vi "Matrix_target.vi"() -> ()   [LabVIEW 2013]
uses:
  <vilib>/Platform/TimedLoop/XDataNode/wakeup.ctl
  <vilib>/Platform/TimedLoop/XDataNode/XDNodeRunTimeDep.lvlib
  <vilib>/Platform/TimedLoop/XDataNode/nitl_modes.ctl
  <vilib>/Platform/TimedLoop/XDataNode/timing_clust.ctl
  <vilib>/Platform/TimedLoop/XDataNode/XDataNode.xnode
  <vilib>/eio/EIONode/EIONode.xnode
  <vilib>/rvi/eio/common/nirviEmuTemplateMethod_errors.vi
  <vilib>/rvi/DataTransferAndStorage/Container/XNode/niFpgaContainer.xnode
  <vilib>/rvi/interface/RandomDataEmulation/nirviRandomDataFpgaReadWriteTemplate.vi
panel:
  out "READ_Number":u64
  in  "RESET":bool
  in  "55":i16
  in  "56":i16
  in  "75":i16
  in  "73":i16
  in  "57":i16=89
  out "String_counter":i16
  in  "String_number":i16
  in  "I2C_Write":bool
  in  "Read2":u8 format="%x"
  in  "Read1":u8 format="%x"
  in  "Device_Read":u8=187 format="%x"
  in  "Reg":u8=9 format="%x"
  in  "Device_Write":u8=186 format="%x"
  in  "91":i16=89
  in  "100_Sclk_divider":i32=25
  out "Sclk":bool
  in  "75_Stop":i16=75
  in  "53":i16=53
  in  "35":i16=35
  in  "17":i16=17
  in  "71":i16=71
  in  "54":i16=54
  in  "36":i16=36
  in  "18":i16=18
  in  "72":i16=72
  in  "50_Rise/Fall divider":i32=50
  in  "0_WE divider":i32
  in  "DataUp":u64
  in  "DataLow":u64
  out "ACK":bool[](array[boolean])
  out "Data_Array":bool[](array[boolean])
  in  "I2C_Request":bool
  in  "FALSE_LV":bool
  in  "FALSE_PIXCLK":bool
  in  "TRUE_FV":bool
  in  "Линия_ прочтена":bool
  in  "Остановите":bool
  out "Линия_готова_на_все":bool
  in  "Читай_Линию":bool
  in  "1_EXTCLK_divider":i16=2
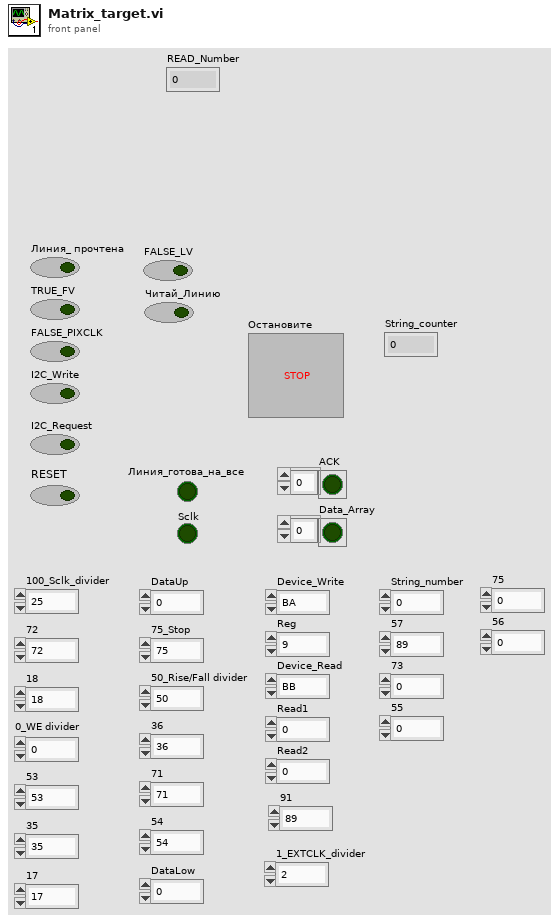
[diagram p1: front panel]
types:
  T1 = typedef "XDNodeRunTimeDep.lvlib/timing_clust.ctl" = cluster{"Expected End [f-1]":u64, "Actual End [f-1]":u64, "Finished Late? [f-1]":bool, "Expected End [i-1]":u64, "Actual End [i-1]":u64, "Finished Late? [i-1]":bool, "Expected Start [i]":u64, "Actual Start [i]":u64, "Expected Start [f]":u64, "Actual Start [f]":u64, "Source Name":string, "Structure Name":string, "Period":i64, "Deadline":i64, "Offset":i64, "Start":i64, "Priority":i32, "Timeout":i32, "Mode":T2, "Wakeup Reason":T3, "Error":errorcluster, "Source Type":string, "Secondary Source Type":string, "Global End Time":u64, "Global Start Time":u64, "Frame Duration":u64, "Iteration Duration":u64, "Assigned CPU":i32, "I/O Scan Engine Mode":u32}
  T2 = typedef "XDNodeRunTimeDep.lvlib/nitl_modes.ctl" = enum32{"No Change", "Process missed periods, maintain original phase", "Discard missed periods, maintain original phase", "Process missed periods, ignore original phase", "Discard missed periods, ignore original phase"}
  T3 = typedef "XDNodeRunTimeDep.lvlib/wakeup.ctl" = enum32{"Normal", "Aborted", "Asynchronous wakeup", "Timing source error", "Timed loop error", "Timeout"}
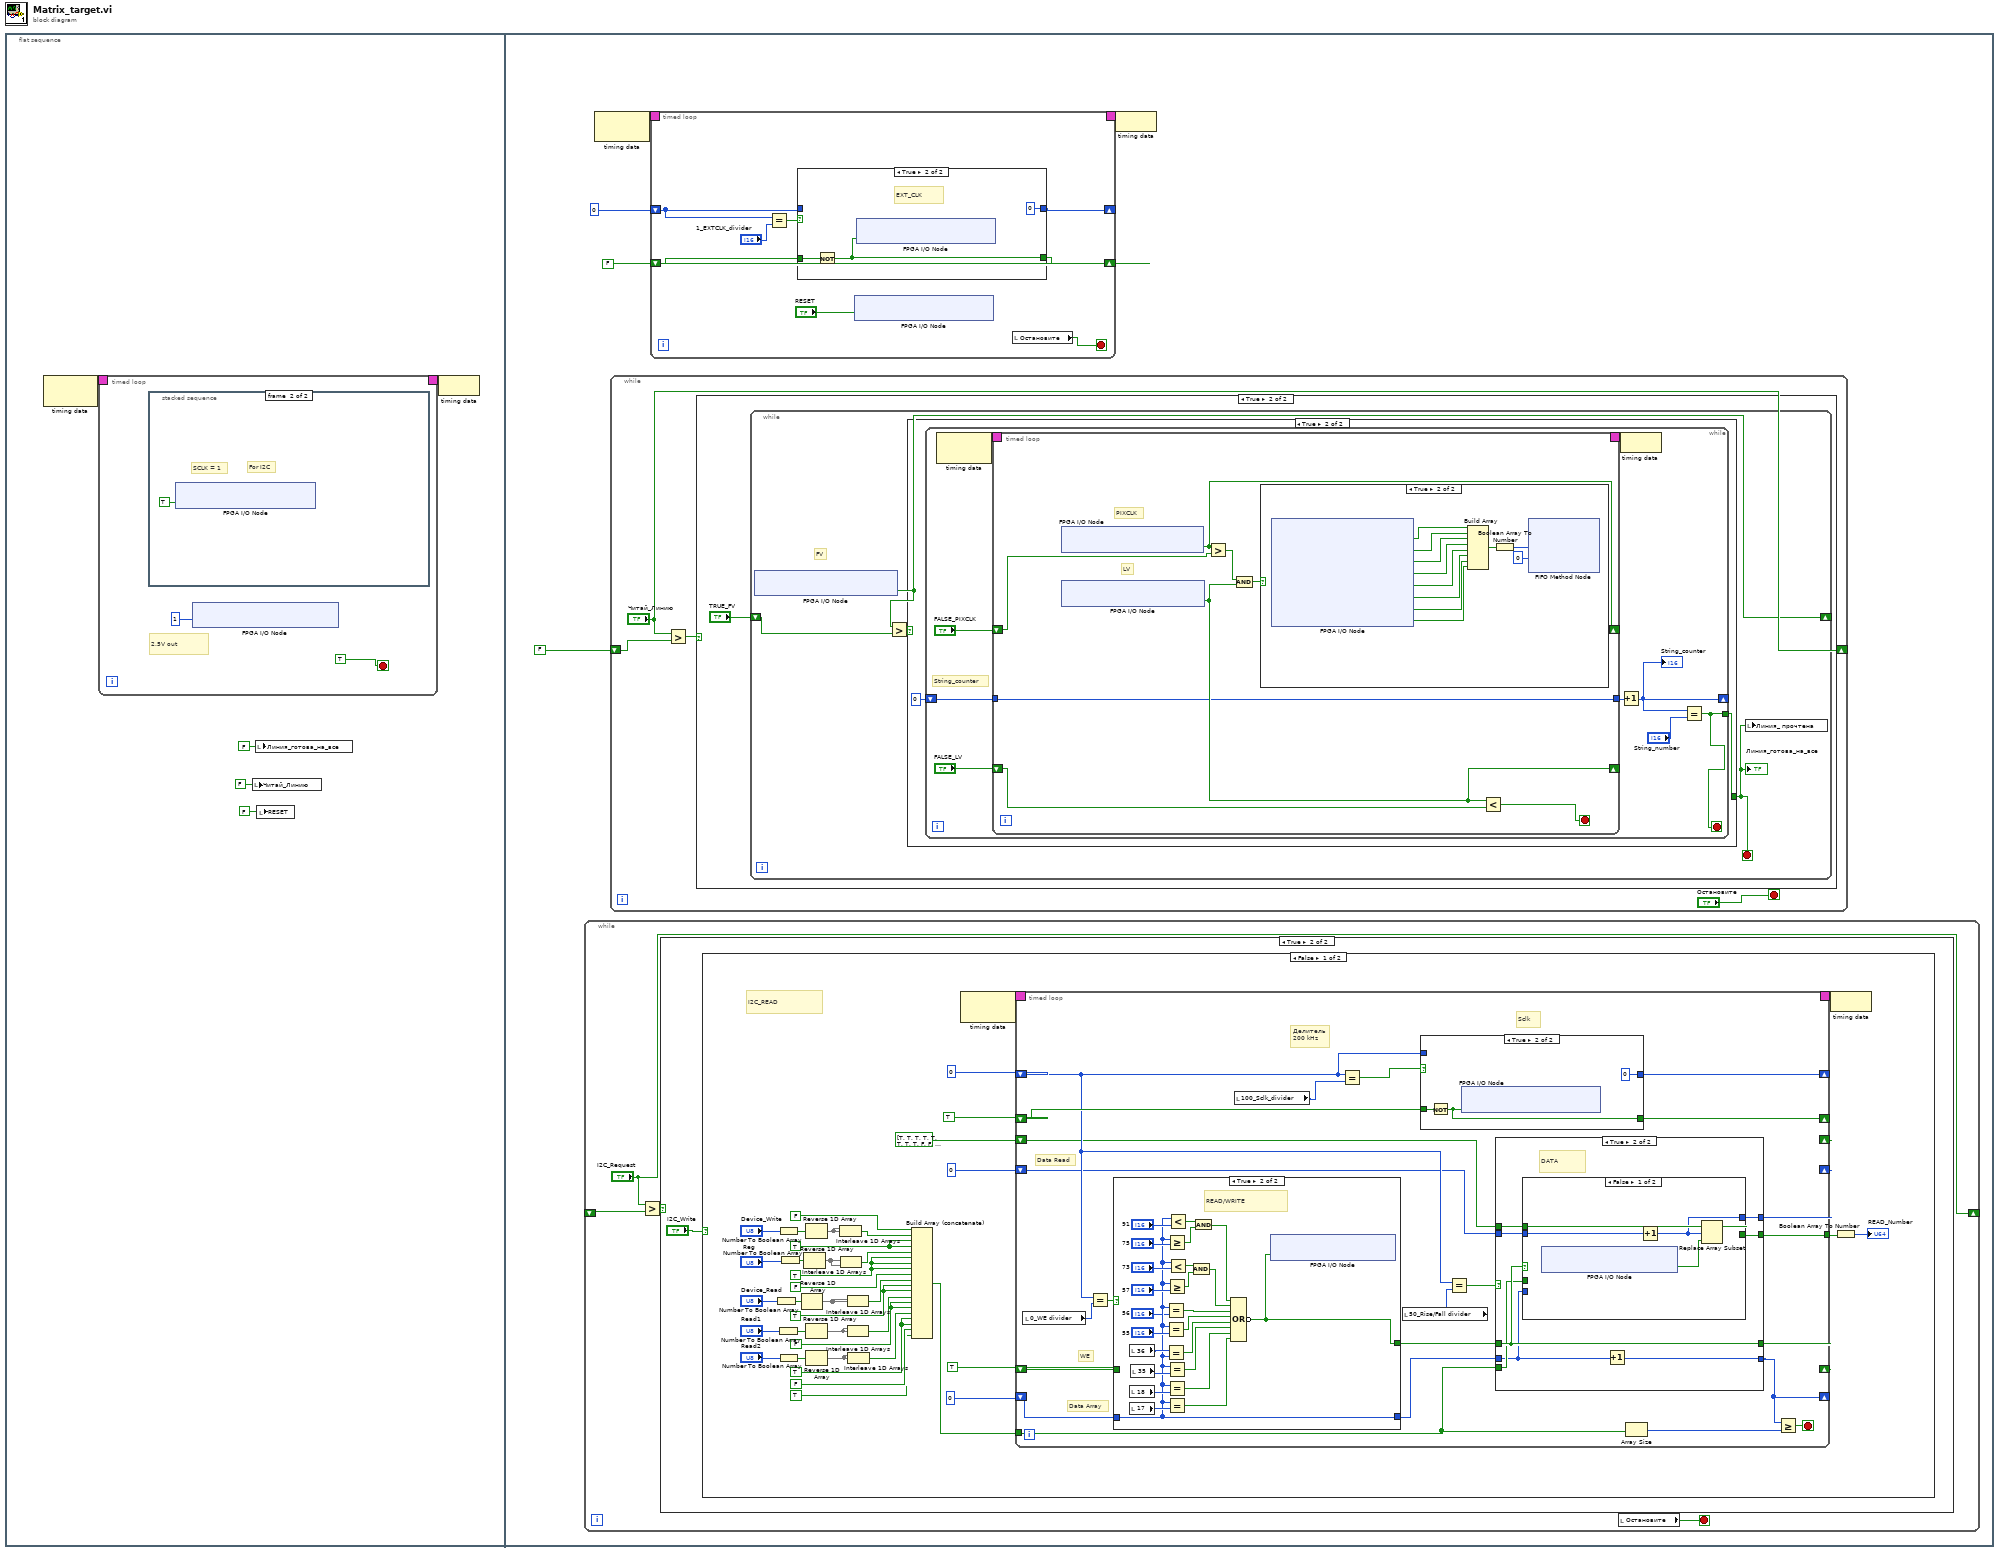
[diagram p0: block diagram]
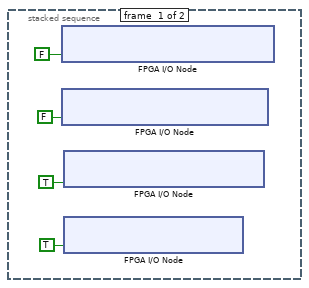
[diagram p2: hidden frame]
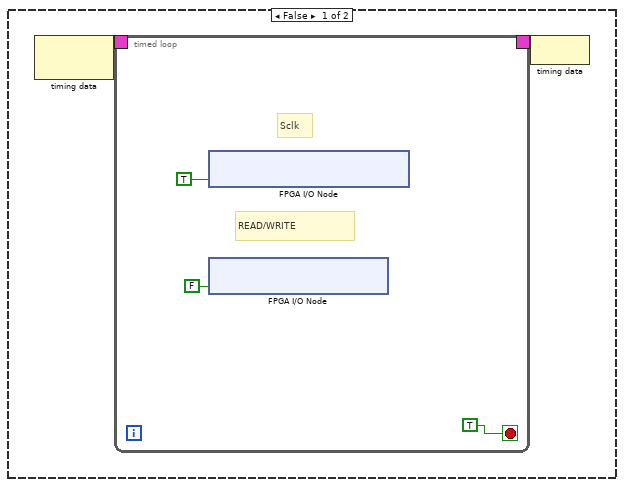
[diagram p3: hidden frame]
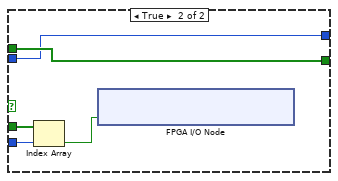
[diagram p6: hidden frame]
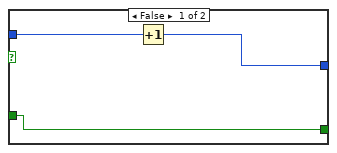
[diagram p7: hidden frame]
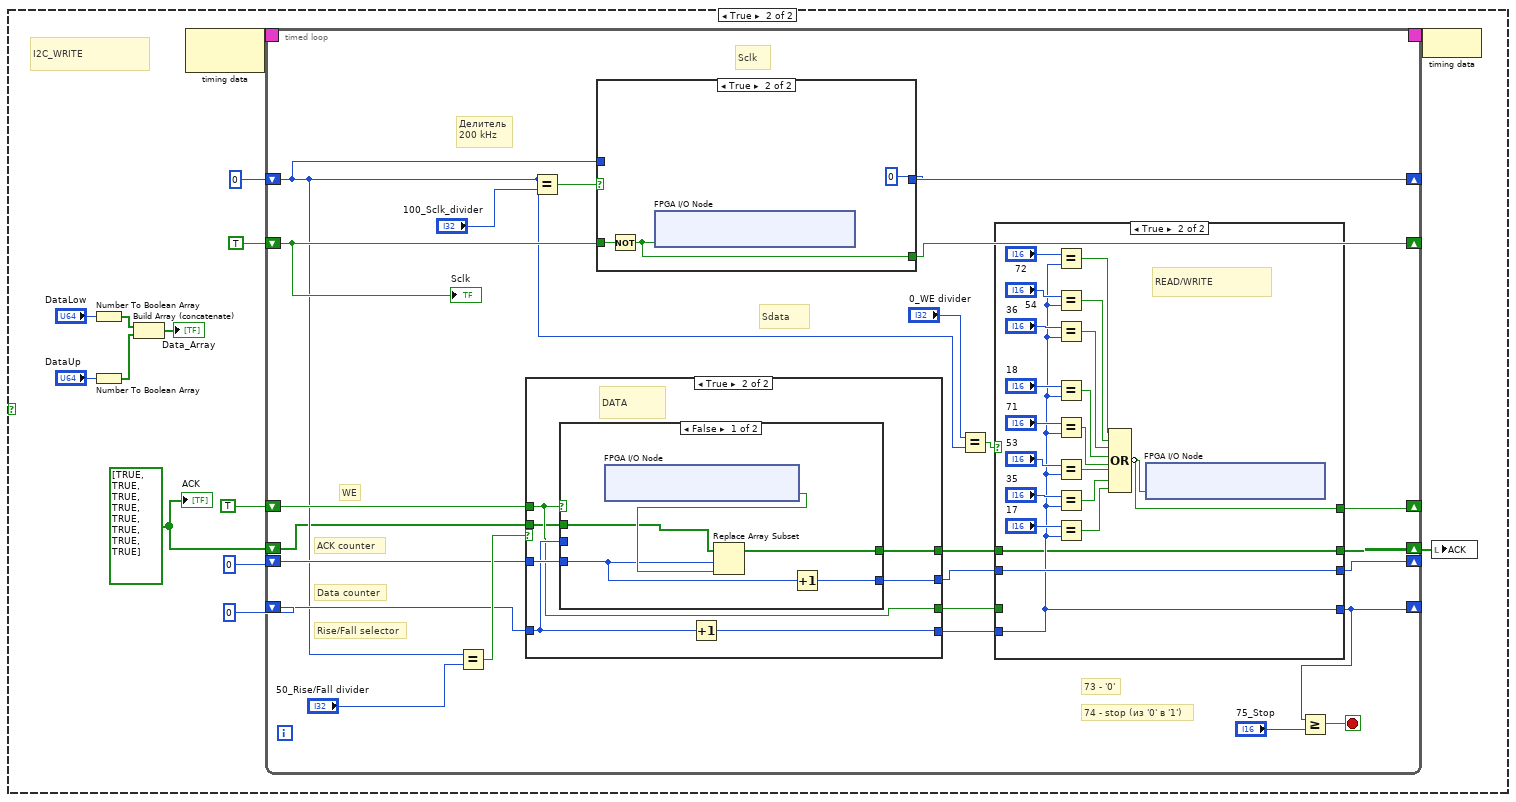
[diagram p8: hidden frame]
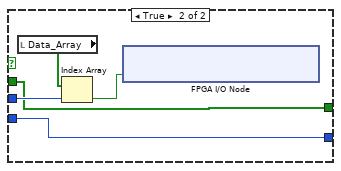
[diagram p11: hidden frame]
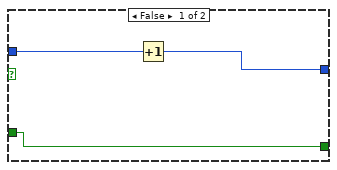
[diagram p12: hidden frame]
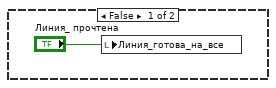
[diagram p13: hidden frame]
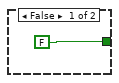
[diagram p14: hidden frame]
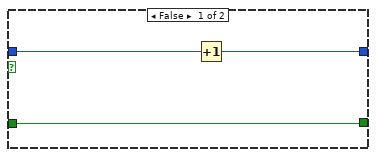
[diagram p16: hidden frame]
diagram:
  n1 = flat-sequence {
    frame #0 {
      n2 = node-c288() -> (w3:T1)  [unwired: 1 in]
      n3 = timed-loop {
        timing: w3 -> [_]
        timing-out: [_] -> w2
        stop <- TRUE stop-if-true
        # "2.5V out"
        n4 = stacked-sequence {
          frame #0 {
            n5 = xnode "FPGA I/O Node"("IO Module\\DDCA_DIO16-23_WE"=FALSE ("IO Module\\DDCA_DIO16-23_WE")) -> ()  [unwired: 1 in, 1 out]
            n6 = xnode "FPGA I/O Node"("IO Module\\DDCA_DIO8-15_WE"=FALSE ("IO Module\\DDCA_DIO8-15_WE")) -> ()  [unwired: 1 in, 1 out]
            n7 = xnode "FPGA I/O Node"("IO Module\\DDCA_DIO0-7_WE"=TRUE ("IO Module\\DDCA_DIO0-7_WE")) -> ()  [unwired: 1 in, 1 out]
            n8 = xnode "FPGA I/O Node"("IO Module\\DDCA_PFI_WE"=TRUE ("IO Module\\DDCA_DIO0-7_WE")) -> ()  [unwired: 1 in, 1 out]
          }
          frame #1 {
            # "For I2C"
            # "SCLK = 1"
            n9 = xnode "FPGA I/O Node"("IO Module\\DDCA_DIO6_Write"=TRUE ("IO Module\\DDCA_DIO6_Write")) -> ()  [unwired: 1 in, 1 out]
          }
        }
        n10 = xnode "FPGA I/O Node"("IO Module\\Local_Supply_Select"=u8 1 ("IO Module\\Local_Supply_Select")) -> ()  [unwired: 1 in, 1 out]
      }
      n11 = local write "Читай_Линию"(FALSE ("Читай_Линию")) -> ()
      n12 = local write "Линия_готова_на_все"(FALSE ("Линия_готова_на_все")) -> ()
      n13 = local write "RESET"(FALSE ("RESET")) -> ()
      n14 = node-c288(w2) -> ()
    }
    frame #1 {
      n15 = while {
        shift-right: ["I2C_Request"] -> _
        shift-left: _ -> [w25]
        stop <- w23 stop-if-true
        n16 = Greater?(x="I2C_Request", y=w25) -> (0:w24:bool)
        n17 = case shown="True" w24 {
          frame False {
            n18 = node-c288() -> (w27:T1)  [unwired: 1 in]
            n19 = timed-loop {
              timing: w27 -> [_]
              timing-out: [_] -> w26
              stop <- TRUE stop-if-true
              # "READ/WRITE"
              # "Sclk"
              n20 = xnode "FPGA I/O Node"("IO Module\\DDCA_DIO6_Write"=TRUE) -> ()  [unwired: 1 in, 1 out]
              n21 = xnode "FPGA I/O Node"("IO Module\\DDCA_PFI_WE"=FALSE ("IO Module\\DDCA_PFI_WE")) -> ()  [unwired: 1 in, 1 out]
            }
            n22 = node-c288(w26) -> ()
          }
          frame True {
            n23 = case shown="False" "I2C_Write" {
              frame False {
                w49 = TRUE
                w51 = FALSE
                w55 = TRUE
                w58 = TRUE
                w61 = TRUE
                # "I2C_READ"
                n24 = Number To Boolean Array(number="Device_Read") -> (Boolean array=w66:bool[])
                n25 = Number To Boolean Array(number="Read1") -> (Boolean array=w46:bool[])
                n26 = Number To Boolean Array(number="Device_Write") -> (Boolean array=w64:bool[])
                n27 = Number To Boolean Array(number="Read2") -> (Boolean array=w45:bool[])
                n28 = Number To Boolean Array(number="Reg") -> (Boolean array=w65:bool[])
                n29 = Reverse 1D Array(array=w66) -> (reversed array=w42:bool[])
                n30 = Reverse 1D Array(array=w65) -> (reversed array=w43:bool[])
                n31 = Reverse 1D Array(array=w64) -> (reversed array=w44:bool[])
                n32 = Reverse 1D Array(array=w46) -> (reversed array=w41:bool[])
                n33 = Reverse 1D Array(array=w45) -> (reversed array=w40:bool[])
                n34 = Interleave 1D Arrays(w44, w44) -> (w62:bool[])
                n35 = Interleave 1D Arrays(w43, w43) -> (w60:bool[])
                n36 = Interleave 1D Arrays(w42, w42) -> (w56:bool[])
                n37 = Interleave 1D Arrays(w41, w41) -> (w52:bool[])
                n38 = Interleave 1D Arrays(w40, w40) -> (w50:bool[])
                n39 = Build Array (concatenate)(FALSE, w62, w61, w61, w60, w58, w58, w58, FALSE, w56, w55, w55, w52, w51, w51, w50, w49, w49, FALSE, TRUE) -> (w59:bool[])
                n40 = node-c288() -> (w75:T1)  [unwired: 1 in]
                n41 = timed-loop {
                  timing: w75 -> [_]
                  timing-out: [_] -> w74
                  shift-right: [w95] -> _
                  shift-left: i16 0 -> [w89]
                  shift-right: [w96] -> _
                  shift-left: TRUE -> [w97]
                  shift-right: [w92] -> _
                  shift-left: TRUE -> [w94]
                  shift-right: [w84] -> _
                  shift-left: i16 0 -> [w88]
                  tunnel: w59 -> [w86]
                  shift-right: [w77] -> _
                  shift-left: bool[] [TRUE, TRUE, TRUE, TRUE, TRUE, TRUE, TRUE, TRUE, FALSE, FALSE, FALSE, FALSE, FALSE, FALSE, FALSE, FALSE, FALSE, FALSE, FALSE, FALSE, FALSE, FALSE, FALSE, FALSE, FALSE, FALSE, FALSE, FALSE, FALSE, FALSE, FALSE, FALSE, FALSE, FALSE, FALSE, FALSE, FALSE, FALSE, FALSE, FALSE, FALSE, FALSE, FALSE, FALSE, FALSE, FALSE, FALSE, FALSE, FALSE, FALSE, FALSE, FALSE, FALSE, FALSE, FALSE, FALSE, FALSE, FALSE, FALSE, FALSE, FALSE, FALSE, FALSE, FALSE] ("ACK") -> [w80]
                  shift-right: [w78] -> _
                  shift-left: i16 0 -> [w79]
                  tunnel: [w77] -> w37
                  stop <- w85 stop-if-true
                  # "Data Read"
                  # "Data Array"
                  # "WE"
                  # "Sclk"
                  # "Делитель\n200 kHz"
                  n42 = local read "0_WE divider"() -> (w81:i32)
                  n43 = Equal?(x=w89, y=w81) -> (x = y?=w91:bool)
                  n44 = case shown="True" w91 {
                    tunnel: [w100 w122] -> w93
                    tunnel: w94 -> [w100 _]
                    tunnel: w88 -> [w99 w102]
                    tunnel: [w99 w102] -> w87
                    frame False {
                    }
                    frame True {
                      # "READ/WRITE"
                      n45 = local read "36"() -> (w113:i16)
                      n46 = local read "18"() -> (w108:i16)
                      n47 = local read "17"() -> (w107:i16)
                      n48 = local read "35"() -> (w104:i16)
                      n49 = Equal?(x=w102, y="56") -> (x = y?=w120:bool)
                      n50 = Equal?(x=w102, y="55") -> (x = y?=w121:bool)
                      n51 = Equal?(x=w113, y=w102) -> (x = y?=w123:bool)
                      n52 = Greater Or Equal?(x=w102, y="75") -> (x >= y?=w116:bool)
                      n53 = Greater Or Equal?(x=w102, y="57") -> (x >= y?=w118:bool)
                      n54 = Equal?(x=w102, y=w104) -> (x = y?=w124:bool)
                      n55 = Equal?(x=w102, y=w108) -> (x = y?=w106:bool)
                      n56 = Equal?(x=w102, y=w107) -> (x = y?=w105:bool)
                      n57 = Less?(x=w102, y="91") -> (x < y?=w115:bool)
                      n58 = Less?(x=w102, y="73") -> (x < y?=w119:bool)
                      n59 = And(x=w119, y=w118) -> (x .and. y?=w117:bool)
                      n60 = And(x=w115, y=w116) -> (x .and. y?=w114:bool)
                      n61 = Compound Arithmetic op=OR(w114, w117, w120, w121, w123, w124, w106, w105) -> (invert w122:bool)
                      n62 = xnode "FPGA I/O Node"("IO Module\\DDCA_PFI_WE"=w122) -> ()  [unwired: 1 in, 1 out]
                    }
                  }
                  n63 = local read "100_Sclk_divider"() -> (w83:i32)
                  n64 = Equal?(x=w89, y=w83) -> (x = y?=w98:bool)
                  n65 = local read "50_Rise/Fall divider"() -> (w82:i32)
                  n66 = case shown="True" w98 {
                    tunnel: [w149 0] -> w95
                    tunnel: w97 -> [w148 w151]
                    tunnel: [w148 w150] -> w96
                    tunnel: w89 -> [w147 _]
                    frame False {
                      n67 = Increment(x=w147) -> (x+1=w149:i32)
                    }
                    frame True {
                      n68 = Not(x=w151) -> (.not. x?=w150:bool)
                      n69 = xnode "FPGA I/O Node"("IO Module\\DDCA_DIO6_Write"=w150) -> ()  [unwired: 1 in, 1 out]
                    }
                  }
                  n70 = Equal?(x=w89, y=w82) -> (x = y?=w90:bool)
                  n71 = case shown="True" w90 {
                    tunnel: w93 -> [w128 w136]
                    tunnel: [w128 w136] -> w92
                    tunnel: w87 -> [w127 w129]
                    tunnel: [w127 w135] -> w84
                    tunnel: w86 -> [_ w134]
                    tunnel: w80 -> [w126 w133]
                    tunnel: [w126 w132] -> w77
                    tunnel: w79 -> [w125 w131]
                    tunnel: [w125 w130] -> w78
                    frame False {
                    }
                    frame True {
                      # "DATA"
                      n72 = case shown="False" w136 {
                        tunnel: w129 -> [_ w146]
                        tunnel: w134 -> [_ w145]
                        tunnel: w133 -> [w141 w143]
                        tunnel: [w140 w143] -> w132
                        tunnel: w131 -> [w138 w142]
                        tunnel: [w139 w142] -> w130
                        frame False {
                          n73 = xnode "FPGA I/O Node"() -> ("IO Module\\DDCA_PFI2_Read"=w137:bool)  [unwired: 1 in, 1 out]
                          n74 = Increment(x=w138) -> (x+1=w139:i16)
                          n75 = Replace Array Subset(array=w141, new element=w137, index=w139) -> (w140:bool[])
                        }
                        frame True {
                          n76 = Index Array(array=w145, index=w146) -> (element=w144:bool)
                          n77 = xnode "FPGA I/O Node"("IO Module\\DDCA_PFI2_Write"=w144) -> ()  [unwired: 1 in, 1 out]
                        }
                      }
                      n78 = Increment(x=w129) -> (x+1=w135:i16)
                    }
                  }
                  n79 = Array Size(array=w86) -> (size(s)=w76:i32)
                  n80 = Greater Or Equal?(x=w84, y=w76) -> (x >= y?=w85:bool)
                }
                n81 = node-c288(w74) -> ()
                n82 = Boolean Array To Number(Boolean array=w37) -> (number=→"READ_Number":u64)
              }
              frame True {
                w157 = bool[] [TRUE, TRUE, TRUE, TRUE, TRUE, TRUE, TRUE, TRUE] ("ACK")
                # "I2C_WRITE"
                n83 = Number To Boolean Array(number="DataLow") -> (Boolean array=w164:bool[])
                n84 = Number To Boolean Array(number="DataUp") -> (Boolean array=w163:bool[])
                n85 = Build Array (concatenate)(w164, w163) -> (→"Data_Array":bool[])
                n86 = node-c288() -> (w170:T1)  [unwired: 1 in]
                n87 = timed-loop {
                  timing: w170 -> [_]
                  timing-out: [_] -> w169
                  shift-right: [w193] -> _
                  shift-left: 0 -> [w182]
                  shift-right: [w192] -> _
                  shift-left: TRUE ("IO Module\\DDCA_DIO0_Write") -> [w189]
                  shift-right: [w179] -> _
                  shift-left: i16 0 -> [w187]
                  shift-right: [w177] -> _
                  shift-left: i16 0 -> [w186]
                  shift-right: [w176] -> _
                  shift-left: TRUE -> [w185]
                  shift-right: [w172] -> w158
                  shift-left: w157 -> [w171]
                  stop <- w174 stop-if-true
                  # "Rise/Fall selector"
                  # "WE"
                  # "Data counter"
                  # "ACK counter"
                  # "74 - stop (из '0' в '1')"
                  # "73 - '0'"
                  # "Sdata"
                  # "Sclk"
                  # "Делитель\n200 kHz"
                  n88 = Equal?(x=w182, y="50_Rise/Fall divider") -> (x = y?=w188:bool)
                  n89 = case shown="True" w188 {
                    tunnel: [w221 w225] -> w180
                    tunnel: w187 -> [w221 w227]
                    tunnel: w186 -> [w222 w229]
                    tunnel: [w222 w228] -> w178
                    tunnel: w185 -> [w220 w226]
                    tunnel: [w220 w226] -> w175
                    tunnel: [w219 w224] -> w173
                    tunnel: w171 -> [w219 w223]
                    frame False {
                    }
                    frame True {
                      # "DATA"
                      n90 = case shown="False" w226 {
                        tunnel: w229 -> [w233 w239]
                        tunnel: [w232 w239] -> w228
                        tunnel: w227 -> [_ w238]
                        tunnel: [w231 w235] -> w224
                        tunnel: w223 -> [w230 w235]
                        frame False {
                          n91 = xnode "FPGA I/O Node"() -> ("IO Module\\DDCA_PFI2_Read"=w234:bool)  [unwired: 1 in, 1 out]
                          n92 = Replace Array Subset(array=w230, new element=w234, index=w233) -> (w231:bool[])
                          n93 = Increment(x=w233) -> (x+1=w232:i16)
                        }
                        frame True {
                          n94 = local read "Data_Array"() -> (w237:bool[])
                          n95 = Index Array(array=w237, index=w238) -> (element=w236:bool)
                          n96 = xnode "FPGA I/O Node"("IO Module\\DDCA_PFI2_Write"=w236) -> ()  [unwired: 1 in, 1 out]
                        }
                      }
                      n97 = Increment(x=w227) -> (x+1=w225:i16)
                    }
                  }
                  n98 = Equal?(x=w182, y="100_Sclk_divider") -> (x = y?=w194:bool)
                  n99 = case shown="True" w194 {
                    tunnel: [w241 0] -> w193
                    tunnel: w182 -> [w242 _]
                    tunnel: w189 -> [w240 w244]
                    tunnel: [w240 w243] -> w192
                    frame False {
                      n100 = Increment(x=w242) -> (x+1=w241:i32)
                    }
                    frame True {
                      n101 = Not(x=w244) -> (.not. x?=w243:bool)
                      n102 = xnode "FPGA I/O Node"("IO Module\\DDCA_DIO6_Write"=w243) -> ()  [unwired: 1 in, 1 out]
                    }
                  }
                  n103 = Equal?(x="0_WE divider", y=w182) -> (x = y?=w181:bool)
                  n104 = case shown="True" w181 {
                    tunnel: w180 -> [w197 w204]
                    tunnel: [w197 w204] -> w179
                    tunnel: [w198 w210] -> w177
                    tunnel: w178 -> [w198 w210]
                    tunnel: [w196 w209] -> w176
                    tunnel: w175 -> [w196 _]
                    tunnel: w173 -> [w195 w199]
                    tunnel: [w195 w199] -> w172
                    frame False {
                    }
                    frame True {
                      # "READ/WRITE"
                      n105 = Equal?(x="72", y=w204) -> (x = y?=w203:bool)
                      n106 = Equal?(x="54", y=w204) -> (x = y?=w200:bool)
                      n107 = Equal?(x="36", y=w204) -> (x = y?=w202:bool)
                      n108 = Equal?(x="18", y=w204) -> (x = y?=w201:bool)
                      n109 = Equal?(x="71", y=w204) -> (x = y?=w211:bool)
                      n110 = Equal?(x="53", y=w204) -> (x = y?=w214:bool)
                      n111 = Equal?(x="35", y=w204) -> (x = y?=w216:bool)
                      n112 = Equal?(x="17", y=w204) -> (x = y?=w218:bool)
                      n113 = Compound Arithmetic op=OR(w203, w200, w202, w201, w211, w214, w216, w218) -> (invert w209:bool)
                      n114 = xnode "FPGA I/O Node"("IO Module\\DDCA_PFI_WE"=w209) -> ()  [unwired: 1 in, 1 out]
                    }
                  }
                  n115 = Greater Or Equal?(x=w179, y="75_Stop") -> (x >= y?=w174:bool)
                  "Sclk" <- w189
                }
                n116 = node-c288(w169) -> ()
                n117 = local write "ACK"(w158) -> ()
                "ACK" <- w157
              }
            }
          }
        }
        n118 = local read "Остановите"() -> (w23:bool)
      }
      n119 = node-c288() -> (w21:T1)  [unwired: 1 in]
      n120 = while {
        shift-right: ["Читай_Линию"] -> _
        shift-left: FALSE -> [w252]
        stop <- "Остановите" stop-if-true
        n121 = Greater?(x="Читай_Линию", y=w252) -> (0:w253:bool)
        n122 = case shown="True" w253 {
          frame False {
            n123 = local write "Линия_готова_на_все"("Линия_ прочтена") -> ()
          }
          frame True {
            n124 = while {
              shift-right: [w257] -> _
              shift-left: "TRUE_FV" -> [w258]
              stop <- w256 stop-if-true
              # "FV"
              n125 = xnode "FPGA I/O Node"() -> ("IO Module\\DDCA_DIO23_Read"=w257:bool)  [unwired: 1 in, 1 out]
              n126 = Greater?(x=w257, y=w258) -> (0:w259:bool)
              n127 = case shown="True" w259 {
                tunnel: [FALSE w262] -> w256
                frame False {
                }
                frame True {
                  n128 = while {
                    tunnel: [w263] -> w262
                    shift-right: [w264] -> _
                    shift-left: i16 0 -> [w266]
                    stop <- w263 stop-if-true
                    # "String_counter"
                    n129 = node-c288() -> (w271:T1)  [unwired: 1 in]
                    n130 = timed-loop {
                      timing: w271 -> [_]
                      timing-out: [_] -> w270
                      shift-right: [w277] -> _
                      shift-left: "FALSE_LV" -> [w278]
                      shift-right: [w273] -> _
                      shift-left: "FALSE_PIXCLK" -> [w274]
                      tunnel: w266 -> [w272]
                      tunnel: [w272] -> w265
                      stop <- w276 stop-if-true
                      # "LV"
                      # "PIXCLK"
                      n131 = xnode "FPGA I/O Node"() -> ("IO Module\\DDCA_DIO17_Read"=w273:bool)  [unwired: 1 in, 1 out]
                      n132 = xnode "FPGA I/O Node"() -> ("IO Module\\DDCA_DIO22_Read"=w277:bool)  [unwired: 1 in, 1 out]
                      n133 = Greater?(x=w273, y=w274) -> (0:w275:bool)
                      n134 = Compound Arithmetic op=AND(w275, w277) -> (w279:bool)
                      n135 = case shown="True" w279 {
                        frame False {
                        }
                        frame True {
                          n136 = xnode "FPGA I/O Node"() -> ("IO Module\\DDCA_DIO8_Read"=w288:bool, "IO Module\\DDCA_DIO9_Read"=w287:bool, "IO Module\\DDCA_DIO10_Read"=w286:bool, "IO Module\\DDCA_DIO11_Read"=w285:bool, "IO Module\\DDCA_DIO12_Read"=w284:bool, "IO Module\\DDCA_DIO13_Read"=w283:bool, "IO Module\\DDCA_DIO14_Read"=w282:bool, "IO Module\\DDCA_DIO15_Read"=w281:bool)  [unwired: 8 in, 8 out]
                          n137 = Build Array(w288, w287, w286, w285, w284, w283, w282, w281) -> (w280:bool[])
                          n138 = Boolean Array To Number(Boolean array=w280) -> (number=w289:u8)
                          n139 = xnode ("FIFO Method Node")("Element"=w289, "Timeout"=0) -> ()  [unwired: 1 in, 2 out]
                        }
                      }
                      n140 = Less?(x=w277, y=w278) -> (x < y?=w276:bool)
                    }
                    n141 = node-c288(w270) -> ()
                    n142 = Increment(x=w265) -> (x+1=w264:i16)
                    "String_counter" <- w264
                    n143 = Equal?(x=w264, y="String_number") -> (x = y?=w263:bool)
                  }
                }
              }
              "Линия_готова_на_все" <- w256
              n144 = local write "Линия_ прочтена"(w256) -> ()
            }
          }
        }
      }
      n145 = timed-loop {
        timing: w21 -> [_]
        timing-out: [_] -> w20
        shift-right: [w297] -> _
        shift-left: i16 0 -> [w299]
        shift-right: [w298] -> _
        shift-left: FALSE -> [w300]
        stop <- w296 stop-if-true
        n146 = Equal?(x=w299, y="1_EXTCLK_divider") -> (x = y?=w302:bool)
        n147 = case shown="True" w302 {
          tunnel: w300 -> [w303 w308]
          tunnel: [w303 w307] -> w298
          tunnel: w299 -> [w305 _]
          tunnel: [w304 i16 0] -> w297
          frame False {
            n148 = Increment(x=w305) -> (x+1=w304:i16)
          }
          frame True {
            # "EXT_CLK"
            n149 = Not(x=w308) -> (.not. x?=w307:bool)
            n150 = xnode "FPGA I/O Node"("IO Module\\DDCA_DIO7_Write"=w307) -> ()  [unwired: 1 in, 1 out]
          }
        }
        n151 = xnode "FPGA I/O Node"("IO Module\\DDCA_DIO5_Write"="RESET") -> ()  [unwired: 1 in, 1 out]
        n152 = local read "Остановите"() -> (w296:bool)
      }
      n153 = node-c288(w20) -> ()
    }
  }
